vi "PS_Testing.vi"() -> ()   [LabVIEW 2012]
uses:
  BotSpeakSubs/BotspeakSettingsUsed.vi
  SubVIs/LVPresent_Globals.vi
panel:
  out "Button":bool
  out "Light":u8(slide) scale=0.0..255.0
  in  "LED":cluster{"Red":bool, "Green":bool, "Blue":bool}
  # "Test the ProtoSnap\n\nTry pushing the button or reading the light sensor.  You can click on any of the areas to see the program that is running"
  # "Click these to turn on LEDs!"
  # "Move your finger over the sensor to see the bar change!"
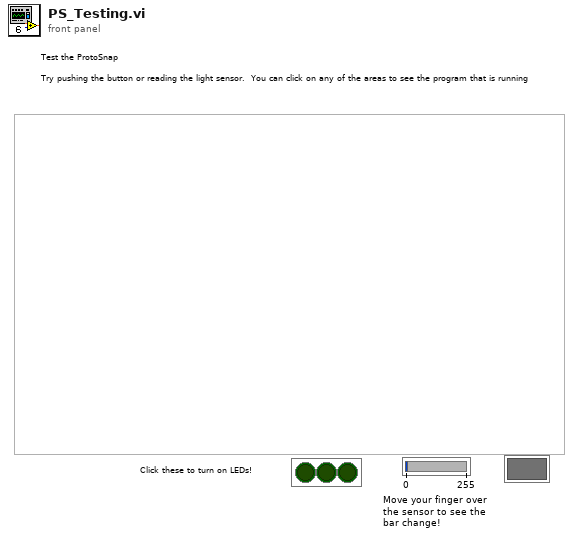
[diagram p1: front panel]
types:
  T1 = typedef "BotSpeak_Control.ctl" = cluster{"Address":string, "Reply EOF":string, "Hardware":string, "Retries":i8, "Timeout":i32, "Open?":bool}
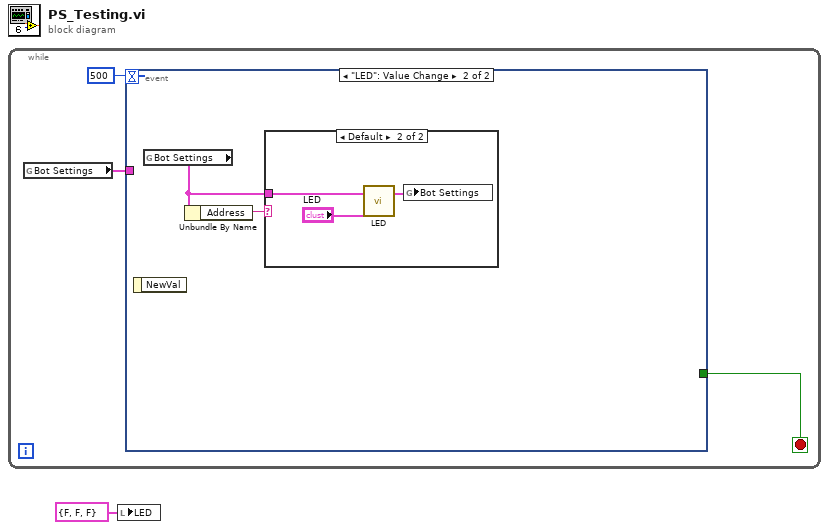
[diagram p0: block diagram]
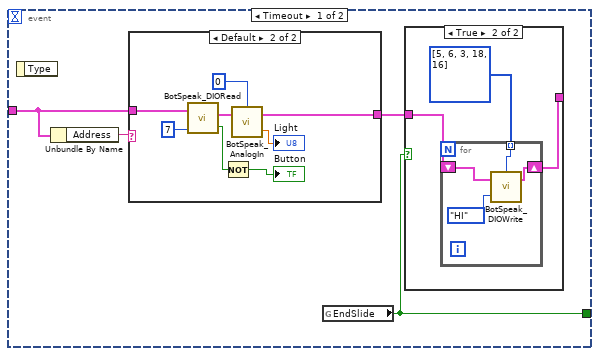
[diagram p2: hidden frame]
diagram:
  n1 = while {
    stop <- w4 stop-if-true
    n2 = global read "BotspeakSettingsUsed.vi" "Bot Settings"() -> (w2:T1)
    n3 = event shown="[1] \"LED\": Value Change" {
      selector: _ -> [_ _]
      dyn-events: _ -> [_ _]
      timeout: 500 -> [_ _]
      tunnel: [w8 _] -> w4
      tunnel: w2 -> [w7 _]
      event Timeout {
        n4 = event-data() -> ()  [unwired: 1 in, 1 out]
        n5 = Unbundle By Name(w7) -> ("Address"=w6:string)
        n6 = case shown="Default" w6 {
          tunnel: w7 -> [w17 w19]
          tunnel: [w17 w18] -> w5
          frame "" {
          }
          frame Default {
            n7 = call <userlib>:"BotSpeak_DIORead.vi"("Bot Settings"=w19, "DIO Line"=u32 7) -> ("State"=w22:bool, "Bot Settings out"=w21:T1)  [unwired: 1 in]
            n8 = Not(x=w22) -> (.not. x?=→"Button":bool)
            n9 = call <userlib>:"BotSpeak_AnalogIn.vi"("Bot Settings"=w21, "A/D Channel"=u8 0) -> ("voltage"=→"Light":dbl, "Bot Settings"=w18:T1)  [unwired: 1 in]
          }
        }
        n10 = global read "LVPresent_Globals.vi" "EndSlide"() -> (w8:bool)
        n11 = case shown="True" w8 {
          tunnel: w5 -> [w9 w11]
          tunnel: [w9 w10] -> _
          frame False {
          }
          frame True {
            n12 = for {
              tunnel: i32[] [5, 6, 3, 18, 16] -> [w16] mode=indexing
              shift-right: [w13] -> w10
              shift-left: w11 -> [w14]
              n13 = call <userlib>:"BotSpeak_DIOWrite.vi"("State"=enum32{"LO", "HI"}."HI", "Bot Settings"=w14, "DIO Line"=w16) -> ("Bot Settings"=w13:T1)  [unwired: 1 out]
            }
          }
        }
      }
      event "LED": Value Change {
        n14 = event-data() -> ()  [unwired: 1 in, 1 out]
        n15 = global read "BotspeakSettingsUsed.vi" "Bot Settings"() -> (w27:T1)
        n16 = Unbundle By Name(w27) -> ("Address"=w26:string)
        n17 = case shown="Default" w26 {
          tunnel: w27 -> [_ w29]
          frame "" {
          }
          frame Default {
            n18 = call "LED.vi"("LED"="LED", "Bot Settings"=w29) -> ("Bot Settings out"=w28:T1)  [unwired: 1 in]
            n19 = global write "BotspeakSettingsUsed.vi" "Bot Settings"(w28) -> ()
          }
        }
      }
    }
  }
  n20 = local write "LED"(cluster{"Red":bool, "Green":bool, "Blue":bool} {"Red"=FALSE, "Green"=FALSE, "Blue"=FALSE} ("LED")) -> ()
